vi "Get Index.vi"(8 "error in (no error)":errorcluster, 11 "Boolean_1D in":refnum<class "Boolean_1D.lvclass">) -> (0 "error out":errorcluster, 2 "Index":i32, 3 "Boolean_1D out":refnum<class "Boolean_1D.lvclass">)   [LabVIEW 2021, in "Boolean_1D.lvclass"]
uses:
  Boolean_1D.lvclass
  Boolean_1D.lvclass/Boolean_1D.ctl
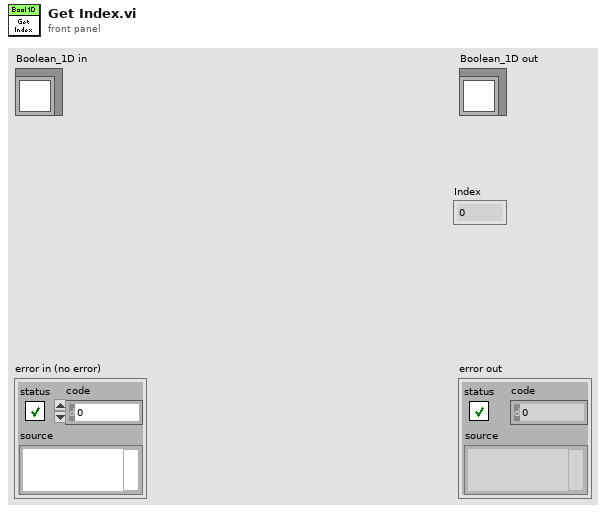
[diagram p1: front panel]
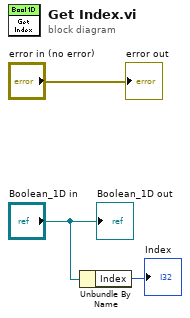
[diagram p0: block diagram]
diagram:
  n1 = Unbundle By Name("Boolean_1D in") -> ("Index"=→"Index":i32)
  "error out" <- "error in (no error)"
  "Boolean_1D out" <- "Boolean_1D in"
